vi "bcp47Name.vi"(8 "Error In":errorcluster, 11 "QLocale In":refnum<class "QLocale.lvclass">) -> (0 "Error Out":errorcluster, 2 "Value":string, 3 "QLocale Out":refnum<class "QLocale.lvclass">)   [LabVIEW 2014, in "QLocale.lvclass"]
doc: "LabVIEW-specific documentation is not yet available. See <b>https://doc.qt.io/qt-5/qlocale.html#bcp47Name</b>"
uses:
  QLocale.lvclass
  LQSerialData/LQSerialData.lvclass/LQSerialData.ctl
  LQ Core.lvlib
  LQSerialData/LQSerialData.lvclass
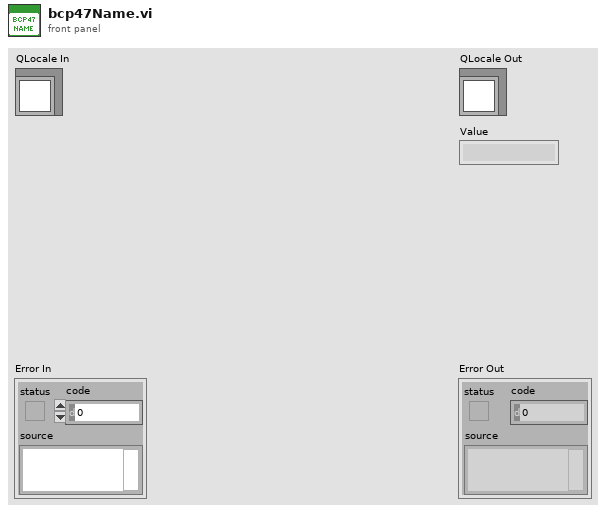
[diagram p1: front panel]
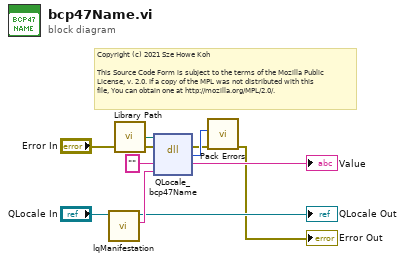
[diagram p0: block diagram]
diagram:
  # "Copyright (c) 2021 Sze Howe Koh\n\nThis Source Code Form is subject to the terms of the Mozilla Public\nLicense, v. 2.0. If a copy of the MPL was not distributed with this\nfile, You can obtain one at http://mozilla.org/MPL/2.0/."
  n1 = call "lqManifestation.vi"("LQSerialData in"="QLocale In") -> ("Manifestation"=w7:string, "LQSerialData out"=→"QLocale Out":refnum<class "QLocale.lvclass">)  [unwired: 9 in]
  n2 = call "Library Path.vi"() -> ("Library Path"=w4:path)
  n3 = dll-call lib="?" fn="QLocale_bcp47Name"(path in=w4, error in="Error In", "_retVal"="" ("retVal"), "_instance"=w7) -> (error out=w2:errorcluster, w3:i32, "_retVal"=→"Value":string)  [unwired: 2 in, 1 out]
  n4 = call "Pack Errors.vi"("Error In"=w2, "Error Code"=w3) -> ("Error Out"=→"Error Out":errorcluster)  [unwired: 9 in]
